vi "excel操作.vi"() -> ()   [LabVIEW 2017]
panel:
  in  "数据":string[][](array[string])
  out "CountRow":i32
  out "Output String":string caption="输出字符串"
  out "Data(Numeral)":sgl[][](array[numeric])
  out "Open":refnum<k7>
  out "Excel.Workbooks":refnum<k7>
  out "添加的数组":dbl[][](array[numeric])
  out "错误输出":errorcluster
  in  "dt":dbl=0.25 format="%0.2f"
  in  "Data Values":dbl[](array[numeric])=[0.0, 1.0, 2.0, 3.0, 4.0, 5.0] caption="数据值" format="%0.2f"
  in  "Excel._Worksheet":refnum<k7>
  in  "ExcelFile":string="D:\\project.xlsx"
  in  "Visible":bool
  in  "Excel._Application":refnum<k7>
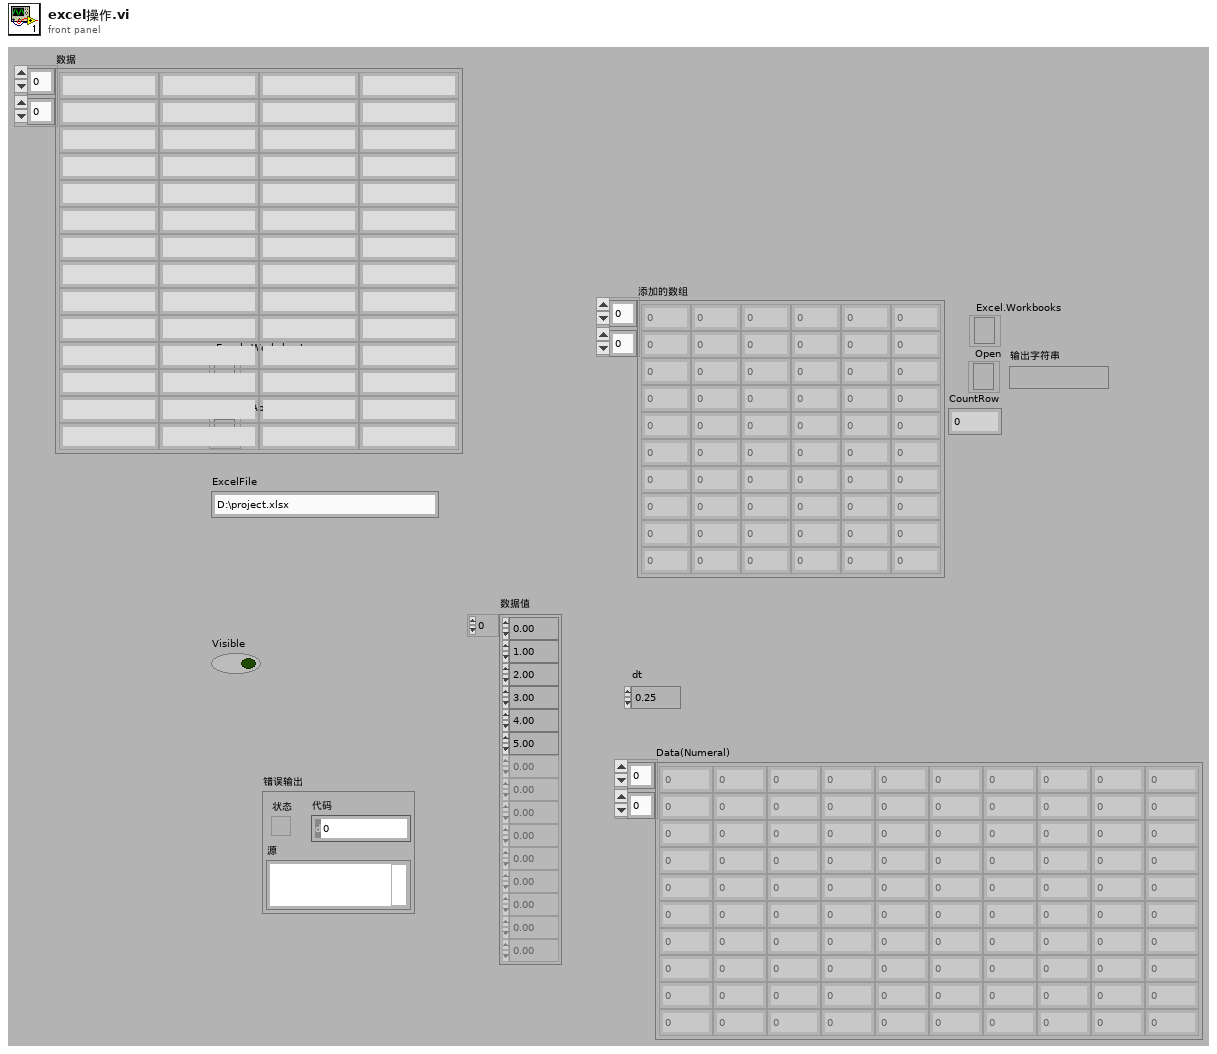
[diagram p1: front panel]
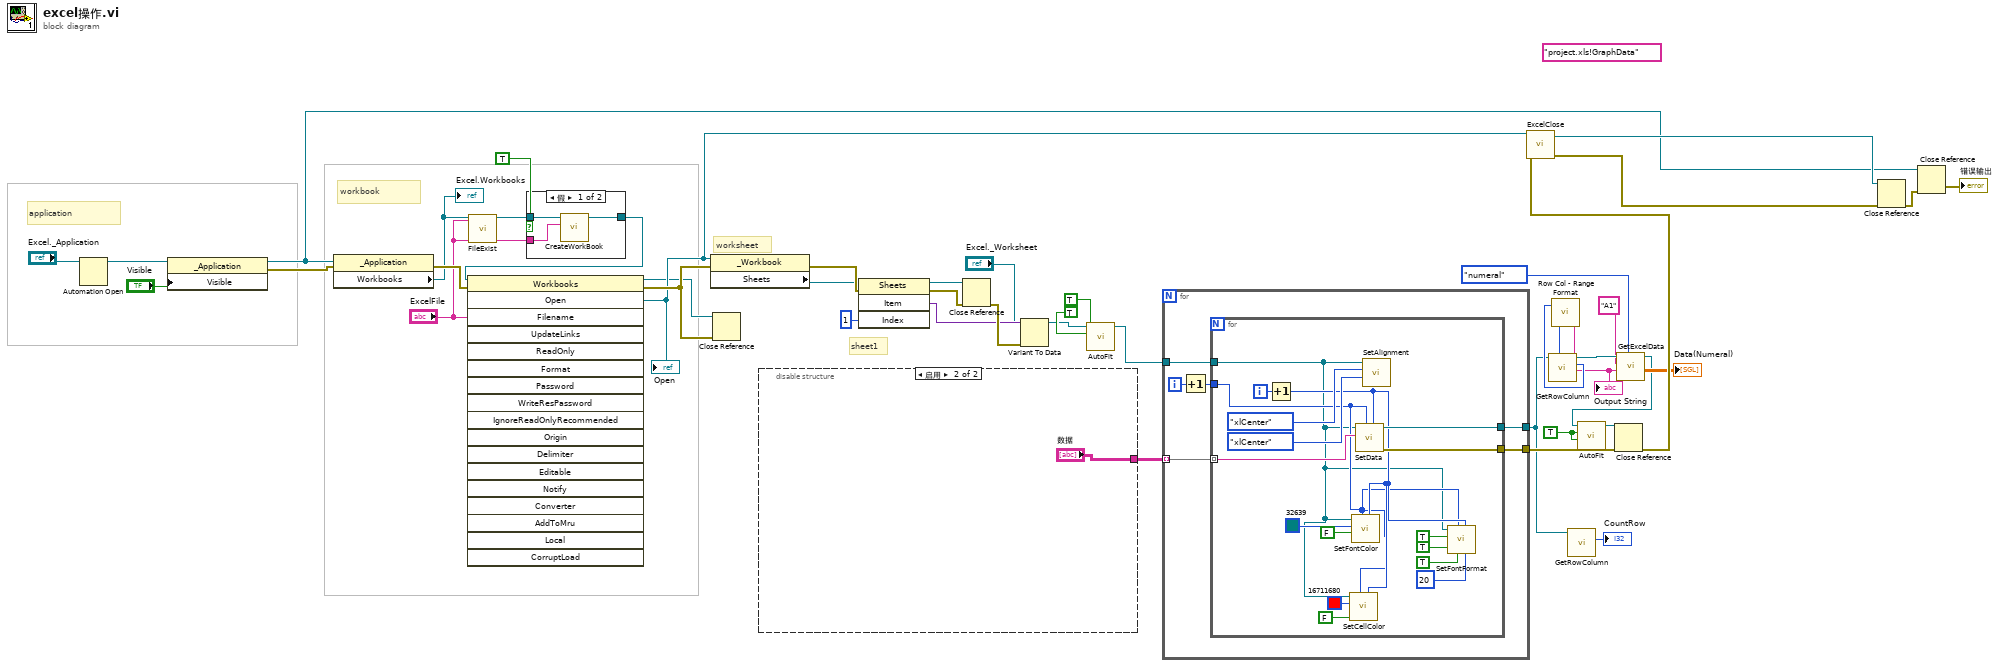
[diagram p0: block diagram]
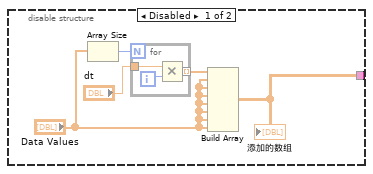
[diagram p2: hidden frame]
diagram:
  w25 = TRUE ("垂直？")
  (unwired) "project.xls!GraphData"
  # "sheet1"
  # "application"
  # "worksheet"
  # "workbook"
  n1 = Automation Open(Automation Refnum="Excel._Application") -> (Automation Refnum=w11:refnum<k7>)  [unwired: 3 in, 1 out]
  n2 = property class="_Application"(reference=w11, "Visible"="Visible") -> (reference out=w8:refnum<k7>, error out=w42:errorcluster)  [unwired: 1 in]
  n3 = property class="_Application"(reference=w8, error in=w42) -> (error out=w43:errorcluster, "Workbooks"=w13:refnum<k7>)  [unwired: 1 out]
  "Excel.Workbooks" <- w13
  n4 = call "FileExist.vi"("FilePath"="ExcelFile") -> ()  [unwired: 9 in, 2 out]
  n5 = case shown="假" TRUE {
    tunnel: w13 -> [w47 w48]
    tunnel: [w46 w48] -> w9
    tunnel: "ExcelFile" -> [w45 _]
    frame False {
      n6 = call "CreateWorkBook.vi"("FileName"=w45, "Excel.Workbooks"=w47) -> ("Excel.Workbooks"=w46:refnum<k7>)  [unwired: 8 in, 1 out]
    }
    frame True {
    }
  }
  n7 = invoke class="Workbooks" method="Open"(reference=w9, error in=w43, "Filename"="ExcelFile") -> (reference out=w10:refnum<k7>, error out=w36:errorcluster, "Open"=w22:refnum<k7>)  [unwired: 15 in, 15 out]
  "Open" <- w22
  n8 = property class="_Workbook"(reference=w22, error in=w36) -> (error out=w37:errorcluster, "Sheets"=w4:refnum<k7>)  [unwired: 1 out]
  n9 = Close Reference(reference=w10, error in (no error)=w36) -> ()  [unwired: 1 out]
  n10 = disable-structure shown="启用" {
    disable-tunnel: [w50 "数据"] -> w35
    frame Disabled {
      n11 = Array Size(array="Data Values") -> (size(s)=w51:i32)
      n12 = for {
        N: w51 -> [_]
        tunnel: "dt" -> [w56]
        tunnel: [w54] -> w52 mode=indexing
        i -> [w55]
        n13 = Multiply(x=w56, y=w55) -> (x*y=w54:dbl)
      }
      n14 = Build Array(w52, "Data Values", "Data Values", "Data Values", "Data Values", "Data Values", "Data Values", "Data Values") -> (w50:dbl[][])
      "添加的数组" <- w50
    }
    frame Enabled {
    }
  }
  n15 = invoke class="Sheets" method="Item"(reference=w4, error in=w37, "Index"=1) -> (reference out=w39:refnum<k7>, error out=w40:errorcluster, "Item"=w23:variant)  [unwired: 1 in, 1 out]
  n16 = Close Reference(reference=w39, error in (no error)=w40) -> (error out=w38:errorcluster)
  n17 = Variant To Data(error in=w38, type="Excel._Worksheet", Variant=w23) -> (data=w2:refnum<k7>)  [unwired: 1 out]
  n18 = call "AutoFit.vi"("水平？"=TRUE, "垂直？"=TRUE ("水平？"), "Excel._Worksheet"=w2) -> ("Excel._Worksheet"=w7:refnum<k7>)  [unwired: 7 in, 1 out]
  n19 = for {
    tunnel: w7 -> [w63]
    tunnel: [w60] -> w6
    tunnel: w35 -> [w59] mode=indexing
    tunnel: [w58] -> w34
    i -> [w62]
    n20 = Increment(x=w62) -> (x+1=w61:i32)
    n21 = for {
      tunnel: w63 -> [w68]
      tunnel: w61 -> [w69]
      tunnel: [w79] -> w60
      tunnel: w59 -> [w77] mode=indexing
      tunnel: [w78] -> w58
      i -> [w80]
      n22 = Increment(x=w80) -> (x+1=w70:i32)
      n23 = call "SetCellColor.vi"("列"=w70, "行"=w69, "取消颜色设置"=FALSE, "颜色盒"=u32 16711680, "Excel._Worksheet"=w68) -> ()  [unwired: 5 in, 2 out]
      n24 = call "SetFontColor.vi"("列"=w70, "行"=w69, "取消字体颜色"=FALSE, "颜色盒"=u32 32639, "Excel._Worksheet"=w68) -> ()  [unwired: 5 in, 2 out]
      n25 = call "SetData.vi"("列"=w70, "行"=w69, "data"=w77, "Excel._Worksheet"=w68) -> ("error out"=w78:errorcluster, "Excel._Worksheet"=w79:refnum<k7>)  [unwired: 6 in]
      n26 = call "SetAlignment.vi"("Vertical Alignment(垂直)"=enum16{"xlTop", "xlCenter", "xlBottom"}."xlCenter", "Horizontal Alignment(水平)"=enum16{"xlRight", "xlLeft", "xlCenter"}."xlCenter", "Excel._Worksheet"=w68) -> ()  [unwired: 7 in, 2 out]
      n27 = call "SetFontFormat.vi"("Size"=20, "列"=w70, "斜体"=TRUE, "行"=w69, "粗体"=TRUE, "下划线"=TRUE, "Excel._Worksheet"=w68) -> ()  [unwired: 3 in, 2 out]
    }
  }
  n28 = call "GetRowColumn.vi"("Excel._Worksheet"=w6) -> ("CountColumn"=w17:i32, "CountRow"=w18:i32, "Excel._Worksheet"=w19:refnum<k7>)  [unwired: 7 in, 1 out]
  n29 = call "Row Col - Range Format.vi"("Column"=w17, "Row"=w18) -> ("Output String"=w16:string)
  "Output String" <- w16
  n30 = call "GetRowColumn.vi"("Excel._Worksheet"=w6) -> ("CountRow"=→"CountRow":i32)  [unwired: 7 in, 3 out]
  n31 = call "GetExcelData.vi"("Format"=enum16{"string", "numeral"}."numeral", "SecondCell"=w16, "FirstCell"="A1", "Excel._Worksheet"=w19) -> ("Data(Numeral)"=→"Data(Numeral)":sgl[][], "Excel._Worksheet"=w14:refnum<k7>)  [unwired: 4 in, 2 out]
  n32 = call "AutoFit.vi"("水平？"=w25, "垂直？"=w25, "Excel._Worksheet"=w14) -> ("Excel._Worksheet"=w26:refnum<k7>)  [unwired: 7 in, 1 out]
  n33 = Close Reference(reference=w26, error in (no error)=w34) -> (error out=w24:errorcluster)
  n34 = call "ExcelClose.vi"("error"=w24, "Excel.Open"=w22) -> ("error out"=w29:errorcluster, "Excel.Open"=w30:refnum<k7>)  [unwired: 8 in]
  n35 = Close Reference(reference=w30, error in (no error)=w29) -> (error out=w32:errorcluster)
  n36 = Close Reference(reference=w8, error in (no error)=w32) -> (error out=→"错误输出":errorcluster)
